vi "VI Tree.vi"   [LabVIEW 2012, in "Phidget Manager.lvlib"]
doc: "${Manager:VITreeHeader}"
uses:
  <instrlib>/Phidgets/Phidget Manager/Phidget Manager.lvlib
panel:
  # "(c) 2015 Phidgets Inc..  ALL RIGHTS RESERVED."
  # "SEE DIAGRAM\nFOR VI TREE."
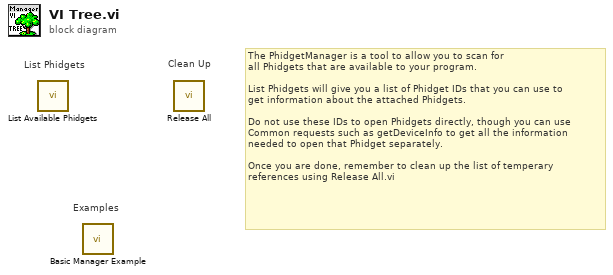
[diagram p0: block diagram]
diagram:
  # "The PhidgetManager is a tool to allow you to scan for\nall Phidgets that are available to your program.\n\nList Phidgets will give you a list of Phidget IDs that you can use to\nget information about the attached Phidgets.\n\nDo not use these IDs to open Phidgets directly, though you can use \nCommon requests such as getDeviceInfo to get all the information\nneeded to open that Phidget separately.\n\nOnce you are done, remember to clean up the list of temperary\nreferences using Release All.vi"
  # "Examples"
  # "Clean Up"
  # "List Phidgets"
  n1 = call <instrlib>:"List Available Phidgets.vi"() -> ()  [unwired: 10 in, 2 out]
  n2 = call <instrlib>:"Basic Manager Example.vi"() -> ()  [unwired: 12 in]
  n3 = call <instrlib>:"Release All.vi"() -> ()  [unwired: 11 in, 1 out]
